vi "SPC_add_data_to_stream.vi"(6 "Buffer":u32[](array[numeric]), 7 "Bytes No":u32, 8 "Error In":errorcluster, 9 "Stream Handle":i16, 11 "DLL Path":path) -> (0 "Error Out":errorcluster, 3 "DLL Path":path)   [LabVIEW 2017]
doc: "The procedure can be used to add photons data to the opened 'buffered' photons stream defined by handle 'stream_hndl'. \nPhotons data in the input buffer can be taken from .spc files or read from module's FIFO.\nData are added to DLL internal buffers which have size between STREAM_MIN_BUF_SIZE and STREAM_MAX_BUF_SIZE. \nInternal buffers are allocated by DLL when required.\nMaximum size of allocated stream buffers is equal STREAM_MAX_SIZE32 for 32-bit DLL and STREAM_MAX_SIZE64 for 64-bit DLL.\nThe buffers are freed, when the stream is closed (SPCM_close_phot_stream) or when, during SPC_get_photons_from_stream call, all photons from the current buffer are extracted ( if an option FREE_BUF_STREAM ( bit 13 in 'stream_type' ) is set). \nProcedure returns error, if 'stream_hndl' is not the handle of the stream opened using SPC_init_buf_stream function.\n\ninfo@becker-hickl.com"
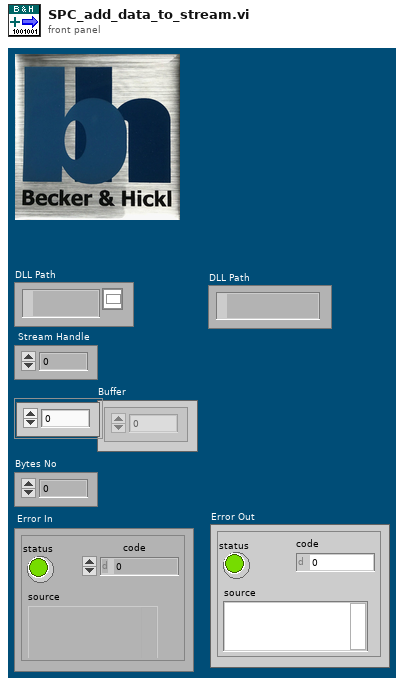
[diagram p1: front panel]
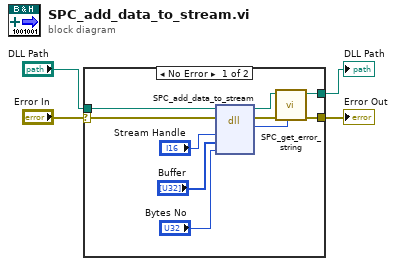
[diagram p0: block diagram]
diagram:
  n1 = case shown="No Error" "Error In" {
    selector: "Error In" -> [w12 w16]
    tunnel: [w10 w16] -> w3
    tunnel: [w6 w15] -> w2
    tunnel: "DLL Path" -> [w9 w15]
    frame No Error {
      n2 = dll-call lib="D:/spcm/lib/lab_view/lv10.0/spcm32.dll" fn="SPC_add_data_to_stream"(path in=w9, error in=w12, "stream_hndl"="Stream Handle", "buffer"="Buffer", "bytes_no"="Bytes No") -> (path out=w7:path, error out=w11:errorcluster, "return type"=w8:i16)  [unwired: 4 in]
      n3 = call "SPC_get_error_string.vi"("ErrorID"=w8, "Error In"=w11, "DLL Path"=w7) -> ("Error Out"=w10:errorcluster, "DLL Path"=w6:path)  [unwired: 6 in, 1 out]
    }
    frame Error {
    }
  }
  "DLL Path" <- w2
  "Error Out" <- w3
